vi "tinySA_example.vi"() -> ()   [LabVIEW 2012]
uses:
  560bf6a7-6959-490f-92d8-cf437f75cecf.vi
  abf36183-ba13-4ef7-a767-6edff4b99444.vi
  9e9068b0-c1ae-4312-b9cc-ba953e1811f6.vi
panel:
  in  "Attenuate (dBm)":u32=10
  in  "auto":bool
  in  "RBW (kHz)":u32=300
  in  "Stop (Hz)":u32=100000000 format="%.0p"
  in  "Start (Hz)":u32 format="%.0p"
  in  "VISAリソース名":refnum<visa-resource-name>="COM21"
  out "Spectrum analyzer":T1(graph)
  in  "停止":bool
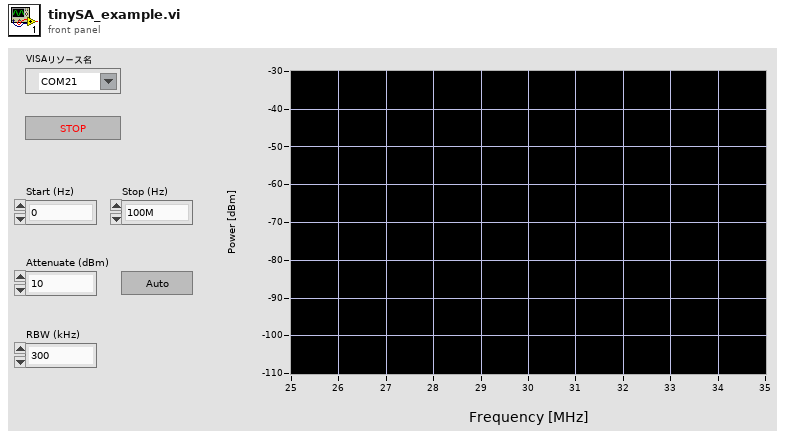
[diagram p1: front panel]
types:
  T1 = cluster{"Frequency (Hz)":dbl[], "Power (dBm)":dbl[]}
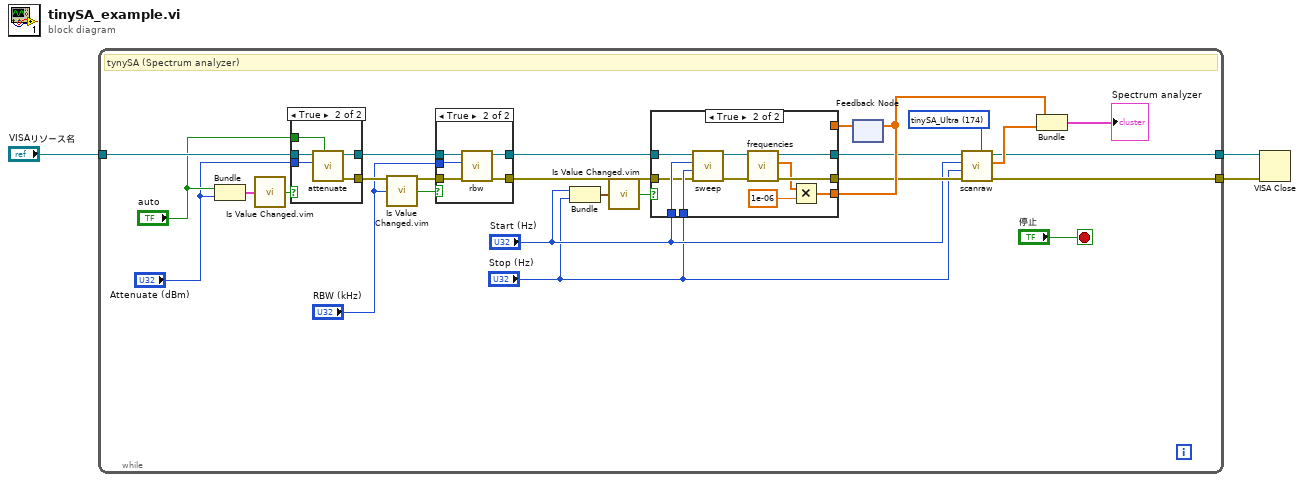
[diagram p0: block diagram]
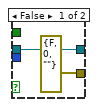
[diagram p2: hidden frame]
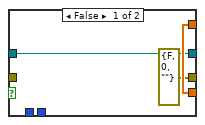
[diagram p4: hidden frame]
diagram:
  n1 = while "Whileループ" {
    tunnel: "VISAリソース名" -> [w12]
    tunnel: [w19] -> w2
    tunnel: [w18] -> w1
    stop <- "停止" stop-if-true
    w28 = u16 174 items=["tinySA"=128, "tinySA_Ultra"=174] ("Offset")
    # "tynySA (Spectrum analyzer)"
    n2 = Bundle("auto"="auto", "Attenuate (dBm)"="Attenuate (dBm)") -> (w5:cluster{"auto":bool, "Attenuate (dBm)":u32})  [unwired: 1 in]
    n3 = call "Is Value Changed.vim"("value"=w5) -> ("changed or first call?"=w4:bool)
    n4 = case shown="TRUE" w4 {
      tunnel: w12 -> [w30 w35]
      tunnel: [w30 w34] -> w11
      tunnel: [errorcluster {"status"=FALSE, "code"=0, "source"=""} ("Error out") w33] -> w10
      tunnel: "auto" -> [_ w32]
      tunnel: "Attenuate (dBm)" -> [_ w31]
      frame False {
      }
      frame True {
        n5 = call "attenuate.vi"("auto"=w32, "Attenuate (dBm)"=w31, "VISA name in"=w35) -> ("Error out"=w33:errorcluster, "VISA name out"=w34:refnum<visa-resource-name>)  [unwired: 7 in]
      }
    }
    n6 = call "Is Value Changed.vim"("value"="RBW (kHz)") -> ("changed or first call?"=w9:bool)
    n7 = case shown="TRUE" w9 {
      tunnel: [w37 w42] -> w14
      tunnel: [w36 w41] -> w13
      tunnel: "RBW (kHz)" -> [_ w40]
      tunnel: w11 -> [w37 w39]
      tunnel: w10 -> [w36 w38]
      frame False {
      }
      frame True {
        n8 = call "rbw.vi"("Error in"=w38, "RBW (kHz)"=w40, "VISA name in"=w39) -> ("Error out"=w41:errorcluster, "VISA name out"=w42:refnum<visa-resource-name>)  [unwired: 7 in]
      }
    }
    n9 = Bundle("Start (Hz)"="Start (Hz)", "Stop (Hz)"="Stop (Hz)") -> (w17:cluster{"Start (Hz)":u32, "Stop (Hz)":u32})  [unwired: 1 in]
    n10 = call "Is Value Changed.vim"("value"=w17) -> ("changed or first call?"=w25:bool)
    n11 = feedback #1() -> (w23:dbl[])  [unwired: 1 in]
    n12 = case shown="TRUE" w25 {
      tunnel: [errorcluster {"status"=FALSE, "code"=0, "source"=""} ("Error out") w56] -> w20
      tunnel: [w44 w55] -> w21
      tunnel: [w45 w54] -> w24
      tunnel: w23 -> [w45 _]
      tunnel: w14 -> [w44 w51]
      tunnel: "Start (Hz)" -> [_ w48]
      tunnel: "Stop (Hz)" -> [_ w47]
      tunnel: w13 -> [_ w46]
      frame False {
      }
      frame True {
        n13 = call "sweep.vi"("Error in"=w46, "Stop (Hz)"=w47, "Start (Hz)"=w48, "VISA name in"=w51) -> ("Error out"=w49:errorcluster, "VISA name out"=w50:refnum<visa-resource-name>)  [unwired: 6 in]
        n14 = call "frequencies.vi"("Error in"=w49, "VISA name in"=w50) -> ("Error out"=w56:errorcluster, "Frequency (Hz)"=w52:dbl[], "VISA name out"=w55:refnum<visa-resource-name>)  [unwired: 7 in]
        n15 = Multiply(x=w52, y=1e-06 ("scale")) -> (x*y=w54:dbl[])
      }
    }
    n16 = feedback-in #1(w24) -> ()
    n17 = call "scanraw.vi"("Offset"=w28, "Error in"=w20, "Stop (Hz)"="Stop (Hz)", "Start (Hz)"="Start (Hz)", "VISA name in"=w21) -> ("Error out"=w18:errorcluster, "Power (dBm)"=w27:dbl[], "VISA name out"=w19:refnum<visa-resource-name>)  [unwired: 4 in]
    n18 = Bundle(w24, "Power (dBm)"=w27) -> (→"Spectrum analyzer":cluster{dbl[], "Power (dBm)":dbl[]})  [unwired: 1 in]
  }
  n19 = VISA Close(VISA resource name=w2, error in (no error)=w1) -> ()  [unwired: 1 out]
